vi "Add Root.vi"(8 "Root Attributes":map{string, string}(c390), 9 "Root Data":string, 10 "New Root Name":string, 11 "Tree Map in":T1) -> (3 "Tree Map Out":T1, 5 "Root Path":string)   [LabVIEW 2020, in "Tree Map.lvlib"]
doc: "Add a root node to Tree Map. This function does not require a valid parent node path. Data asociated with this node can be optionally specified.\n\n<b>NOTE</b> Be careful not to use XML special characters for the data or name of the node if you intend to flatten and unflatten from XML. This can cause error in XML functions.\n\n<b>Author:</b> Piotr Kruczkowski <PrimaryKey>\n<b>License:</b> NewBSD\n\nCopyright (c) 2019, National Instruments\nAll rights reserved.\n\nRedistribution and use in source and binary forms, with or without\nmodification, are permitted provided that the following conditions are met:\n1. Redistributions of source code must retain the above copyright\n notice, this list of conditions and the following disclaimer.\n2. Redistributions in binary form must reproduce the above copyright\n notice, this list of conditions and the following disclaimer in the\n documentation and/or other materials provided with the distribution.\n3. Neither the name of National Instruments nor the\n names of its contributors may be used to endorse or promote products\n derived from this software without specific prior written permission.\n\nTHIS SOFTWARE IS PROVIDED BY National Instruments ''AS IS'' AND ANY\nEXPRESS OR IMPLIED WARRANTIES, INCLUDING, BUT NOT LIMITED TO, THE IMPLIED\nWARRANTIES OF MERCHANTABILITY AND FITNESS FOR A PARTICULAR PURPOSE ARE\nDISCLAIMED. IN NO EVENT SHALL National Instruments BE LIABLE FOR ANY\nDIRECT, INDIRECT, INCIDENTAL, SPECIAL, EXEMPLARY, OR CONSEQUENTIAL DAMAGES\n(INCLUDING, BUT NOT LIMITED TO, PROCUREMENT OF SUBSTITUTE GOODS OR SERVICES;\nLOSS OF USE, DATA, OR PROFITS; OR BUSINESS INTERRUPTION) HOWEVER CAUSED AND\nON ANY THEORY OF LIABILITY, WHETHER IN CONTRACT, STRICT LIABILITY, OR TORT\n(INCLUDING NEGLIGENCE OR OTHERWISE) ARISING IN ANY WAY OUT OF THE USE OF THIS\nSOFTWARE, EVEN IF ADVISED OF THE POSSIBILITY OF SUCH DAMAGE."
uses:
  Tree Map.lvlib
  Tree Map Data.ctl
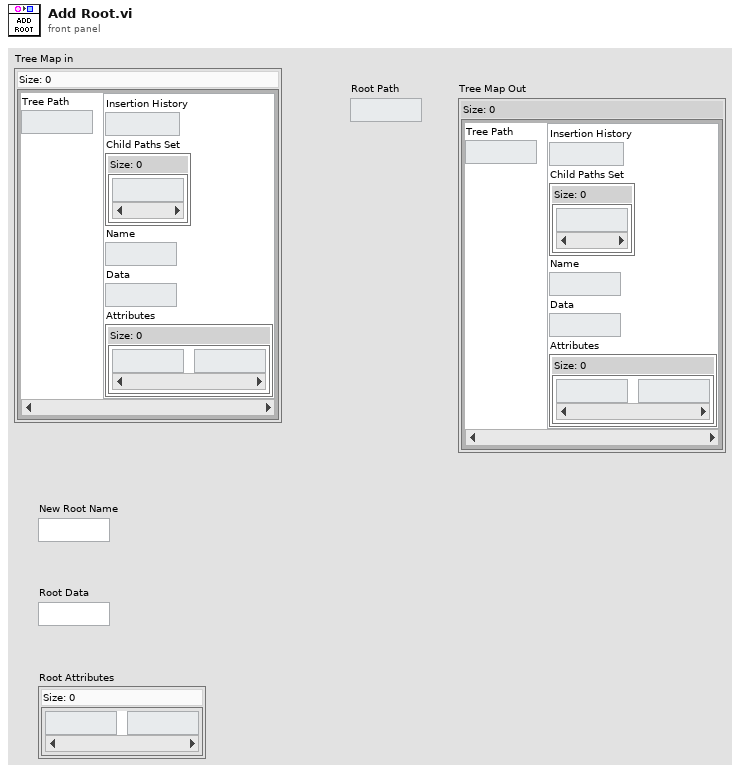
[diagram p1: front panel]
types:
  T1 = typedef "Tree Map.lvlib/Tree Map Data.ctl" = map{string, cluster{"Insertion History":i32, "Child Paths Set":set{string}, "Name":string, "Data":string, "Attributes":map{string, string}}}
  T2 = cluster{"Insertion History":i32, "Child Paths Set":set{string}, "Name":string, "Data":string, "Attributes":map{string, string}}
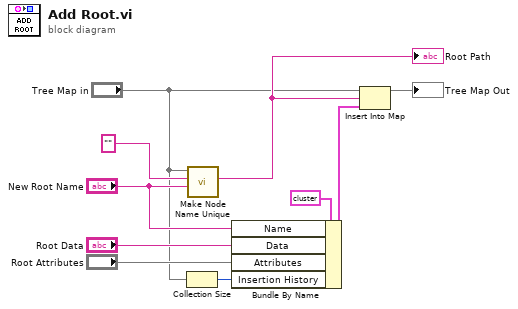
[diagram p0: block diagram]
diagram:
  n1 = Collection Size(1:"Tree Map in") -> (0:w1:i32)
  n2 = call "Make Node Name Unique.vi"("New Node Name"="New Root Name", "Parent Path"="", "Tree Map In"="Tree Map in") -> ("Node Path"=w6:string)  [unwired: 8 in]
  "Root Path" <- w6
  n3 = Bundle By Name(cluster=T2 {"Insertion History"=0, "Child Paths Set"={}, "Name"="", "Data"="", "Attributes"={}} ("Node"), "Name"="New Root Name", "Data"="Root Data", "Attributes"="Root Attributes", "Insertion History"=w1) -> (w7:T2)
  n4 = Insert Into Map(map in="Tree Map in", key=w6, value=w7) -> (map out=→"Tree Map Out":T1)  [unwired: 2 out]
